vi "String_2_Number.vi"(1 "Value":string) -> (0 "Numeric":dbl)   [LabVIEW 2010]
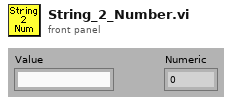
[diagram p1: front panel]
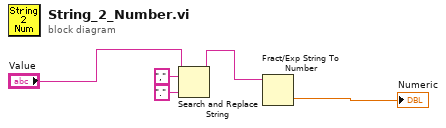
[diagram p0: block diagram]
diagram:
  n1 = Search and Replace String(input string="Value", search string=",", replace string="." ("replace string (\"\")")) -> (result string=w5:string)  [unwired: 5 in, 3 out]
  n2 = Fract/Exp String To Number(string=w5) -> (number=→"Numeric":dbl)  [unwired: 4 out]
